vi "XIPIN_3GPP2_Turbo_Encoder_2_0.vi"   [LabVIEW 2017]
doc: "Rev 1. The Turbo encoder LogiCORE from Xilinx is a high-speed, compact Turbo Convolutional Encoder which meets the 3GPP2 C.S0024-B specification. The core is delivered through the Xilinx CORE Generator System and integrates seamlessly with the Xilinx design flow.\n------------------------------------\n<b>Need License</b> : Yes"
uses:
  <vilib>/rvi/XilinxIP/XIPIN_XNode/niFpgaXIPIN.xnode
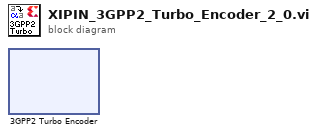
[diagram p0: block diagram]
diagram:
  n1 = xnode ("3GPP2 Turbo Encoder")() -> ()
